vi "Scanner Action-Status.vi"(8 "error in (no error)":errorcluster, 10 "Message Data":variant, 11 "Data Cluster":T1={"Link"={"Connection"=enum."USB", "Host or IP address (TCP/IP)"="", "Port (Serial/USB)"="COM1"}, "VISA resource"="", "Writer Queue"=refnum, "Status"=FALSE}) -> (0 "error out":errorcluster, 3 "Data Cluster out":T1={"Link"={"Connection"=enum."USB", "Host or IP address (TCP/IP)"="", "Port (Serial/USB)"="COM1"}, "VISA resource"="", "Writer Queue"=refnum, "Status"=FALSE})   [LabVIEW 2020, in "Hiden Scanner.lvlib"]
uses:
  Hiden Scanner.lvlib
  Scanner Hardware Configuration.ctl
  support/Message Queue/Message Cluster.ctl
  support/Message Queue/Message Queue.lvlib
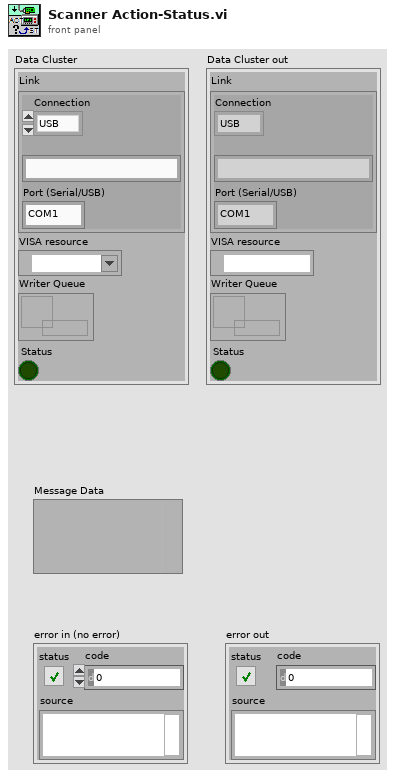
[diagram p1: front panel]
types:
  T1 = typedef "Hiden Scanner.lvlib/Scanner Hardware Configuration.ctl" = cluster{"Link":cluster{"Connection":enum16{"Serial", "TCP/IP", "USB"}, "Host or IP address (TCP/IP)":string, "Port (Serial/USB)":string}, "VISA resource":refnum<visa-resource-name>, "Writer Queue":refnum<queue>, "Status":bool}
  T2 = typedef "Message Queue.lvlib/Message Cluster.ctl" = cluster{"Message":string, "Message Data":variant}
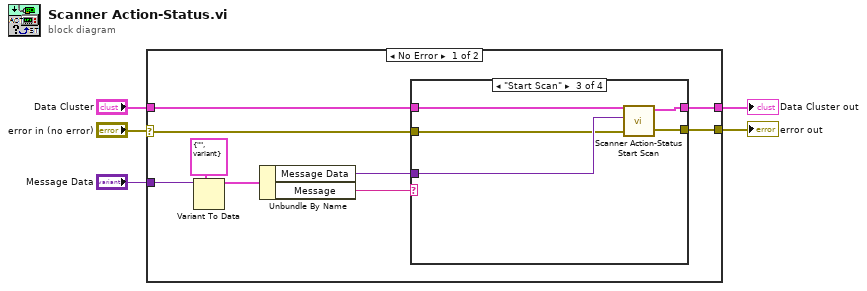
[diagram p0: block diagram]
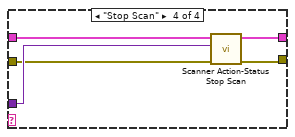
[diagram p4: hidden frame]
diagram:
  n1 = case shown="No Error" "error in (no error)" {
    selector: "error in (no error)" -> [w7 w29]
    tunnel: [w14 w29] -> w5
    tunnel: "Data Cluster" -> [w13 w30]
    tunnel: [w12 w30] -> w3
    tunnel: "Message Data" -> [w8 _]
    frame No Error {
      n2 = Variant To Data(type=T2 {"Message"="", "Message Data"=variant} ("element"), Variant=w8) -> (data=w10:T2)  [unwired: 1 in, 1 out]
      n3 = Unbundle By Name(w10) -> ("Message Data"=w6:variant, "Message"=w11:string)
      n4 = case shown="\"Start Scan\"" w11 {
        tunnel: w6 -> [_ _ w22 w26]
        tunnel: [w16 w18 w21 w27] -> w12
        tunnel: w13 -> [w16 w18 w23 w28]
        tunnel: w7 -> [w15 w17 w19 w25]
        tunnel: [w15 w17 w20 w24] -> w14
        frame "False", Default {
        }
        frame "Calibrate Axes" {
        }
        frame "Start Scan" {
          n5 = call "Scanner Action-Status Start Scan.vi"("error in (no error)"=w19, "Message Data"=w22, "Data Cluster in"=w23) -> ("error out"=w20:errorcluster, "Data Cluster out"=w21:T1)  [unwired: 7 in]
        }
        frame "Stop Scan" {
          n6 = call "Scanner Action-Status Stop Scan.vi"("error in (no error)"=w25, "Message Data"=w26, "Data Cluster in"=w28) -> ("error out"=w24:errorcluster, "Data Cluster out"=w27:T1)  [unwired: 7 in]
        }
      }
    }
    frame Error {
    }
  }
  "error out" <- w5
  "Data Cluster out" <- w3
